vi "HeaderAction.vi"(0 "InstrClass":refnum<class "KlingerMotor.lvclass"> caption="DNL_LabVIEW Object in", 11 "error in (no error)":errorcluster caption="entrée d'erreur (pas d'erreur)") -> (4 "InstrClassOut":refnum<class "KlingerMotor.lvclass"> caption="DNL_LabVIEW Object out", 6 "DataNames":string[](array[string]), 8 "Instr Name":string, 10 "HeaderString":string, 14 "DisplayNames":string[](array[string]), 15 "error out":errorcluster caption="sortie d'erreur")   [LabVIEW 2012, in "KlingerMotor.lvclass"]
uses:
  KlingerMotor.lvclass
  KlingerMotor.lvclass/KlingerMotor.ctl
  <userlib>/KlingerV2/KlingerV2 Params.ctl
  BaseDevice/BaseDevice.lvclass
panel:
  in  "Type":i32(ring) items=["UE30", "UE72"]
  in  "Axe":u8(ring)=3 items=["W", "X", "Y", "Z"]
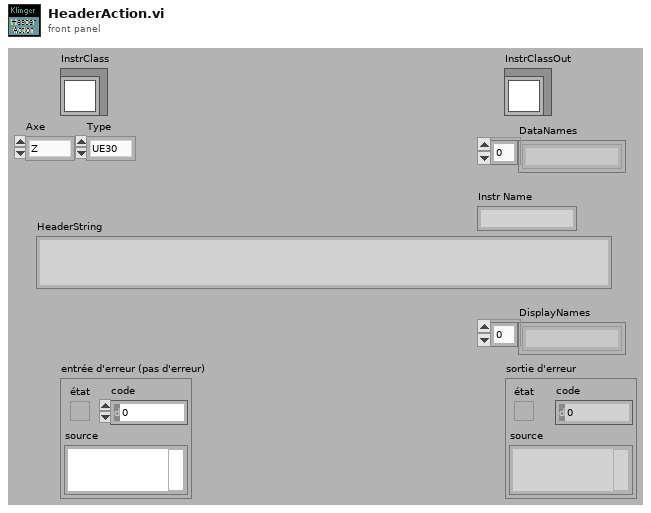
[diagram p1: front panel]
types:
  T1 = typedef "KlingerV2 Params.ctl" = enum16{"Type", "Origine", "Encodeur", "TypeMouv", "FactConv", "Nom", "CorrParams", "KlingCtrlPar", "Speed", "Acc", "Avance", "Tous"}
  T2 = typedef "KlingerMotor.lvclass/KlingerMotor_Func.ctl" = enum16{"Positions (mm)", "ReadWPos (ps)", "ReadZPos (ps)"}
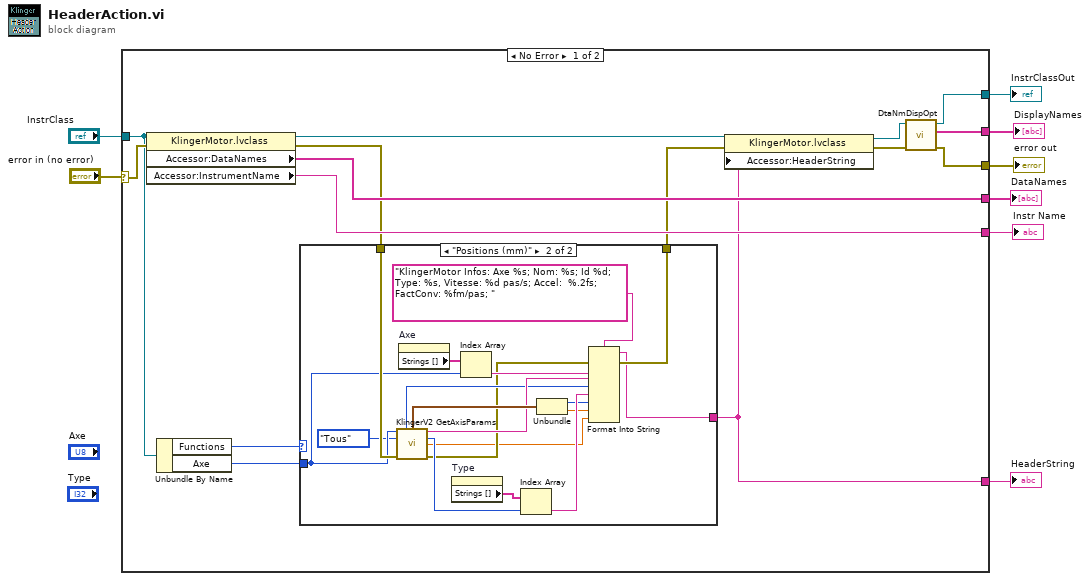
[diagram p0: block diagram]
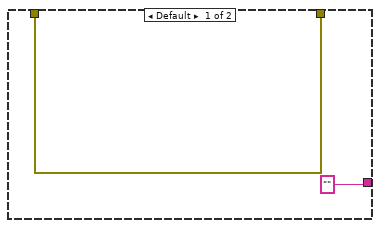
[diagram p2: hidden frame]
diagram:
  n1 = case shown="No Error" "error in (no error)" {
    selector: "error in (no error)" -> [w23 w44]
    tunnel: [w17 _] -> w7
    tunnel: [w22 _] -> w6
    tunnel: "InstrClass" -> [w19 w45]
    tunnel: [w15 w44] -> w4
    tunnel: [w14 w45] -> w2
    tunnel: [w20 _] -> w3
    tunnel: [w12 _] -> w1
    frame No Error {
      n2 = property class="KlingerMotor.lvclass"(reference=w19, error in=w23) -> (reference out=w21:refnum<class "KlingerMotor.lvclass">, error out=w11:errorcluster, "Accessor:DataNames"=w22:string[], "Accessor:InstrumentName"=w20:string)
      n3 = Unbundle By Name(w19) -> ("Functions"=w18:T2, "Axe"=w10:u8)
      n4 = case shown="\"Positions (mm)\"" w18 {
        tunnel: ["" ("HeaderString") w27] -> w17
        tunnel: w11 -> [w24 w43]
        tunnel: w10 -> [_ w41]
        tunnel: [w24 w29] -> w9
        frame Default {
        }
        frame "Positions (mm)" {
          n5 = call <userlib>:"KlingerV2 GetAxisParams.vi"("Axe"=w41, "Param"=KlingerV2_Params."Tous", "error in"=w43) -> ("ID Number"=w36:i32, "Speed"=w39:cluster{"Vitesse":i32, "Accel":dbl}, "Nom de l'axe"=w37:string, "Type"=w34:i32, "FactConv"=w26:dbl, "error out"=w30:errorcluster)  [unwired: 3 in, 4 out]
          n6 = property on="Axe" class="Ring (strict)"() -> ("Strings []"=w42:string[])  [unwired: 2 in, 2 out]
          n7 = property on="Type" class="Ring (strict)"() -> ("Strings []"=w35:string[])  [unwired: 2 in, 2 out]
          n8 = Index Array(array=w42, index=w41) -> (element=w38:string)
          n9 = Index Array(array=w35, index=w34) -> (element=w33:string)
          n10 = Unbundle(w39) -> ("Vitesse"=w32:i32, "Accel"=w31:dbl)
          n11 = Format Into String(format string="KlingerMotor Infos: Axe %s; Nom: %s; Id %d; Type: %s, Vitesse: %d pas/s; Accel:  %.2fs; FactConv: %fm/pas; ", error in=w30, w38, w37, w36, w33, w32, w31, w26) -> (resulting string=w27:string, error out=w29:errorcluster)  [unwired: 1 in]
        }
      }
      n12 = property class="KlingerMotor.lvclass"(reference=w21, error in=w9, "Accessor:HeaderString"=w17) -> (reference out=w13:refnum<class "KlingerMotor.lvclass">, error out=w16:errorcluster)
      n13 = call "DtaNmDispOpt.vi"("error in (no error)"=w16, "BaseDevice en entrée"=w13) -> ("error out"=w15:errorcluster, "DisplayNames"=w12:string[], "BaseDevice en sortie"=w14:refnum<class "KlingerMotor.lvclass">)  [unwired: 7 in]
    }
    frame Error {
    }
  }
  "error out" <- w4
  "InstrClassOut" <- w2
  "DataNames" <- w6
  "HeaderString" <- w7
  "Instr Name" <- w3
  "DisplayNames" <- w1
